vi "ASDA-A2_Release.vi"(8 "error in":errorcluster, 11 "Buffer Data":T1) -> (0 "error out":errorcluster)   [LabVIEW 2016]
uses:
  Data Def/ASDA-A2_Buffer Data.ctl
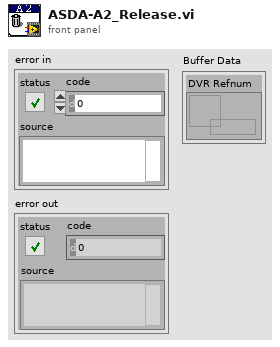
[diagram p1: front panel]
types:
  T1 = typedef "ASDA-A2_Buffer Data.ctl" = cluster{"DVR Refnum":refnum<data-value>}
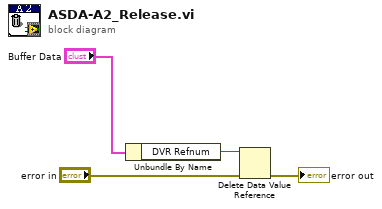
[diagram p0: block diagram]
diagram:
  n1 = Unbundle By Name("Buffer Data") -> ("DVR Refnum"=w3:refnum<data-value>)
  n2 = Delete Data Value Reference(data value reference=w3, error in="error in") -> (error out=→"error out":errorcluster)  [unwired: 1 out]
